vi "F Dwf Enum.vi"(8 "error in (no error)":errorcluster, 10 "pcDevice":i32, 11 "enumfilter":i32) -> (0 "error out":errorcluster, 2 "pcDevice out":i32, 3 "function return":i32)   [LabVIEW 2024, in "Olasdwf.lvlib"]
doc: "DWFAPI int FDwfEnum(ENUMFILTER enumfilter, int *pcDevice);"
uses:
  Olasdwf.lvlib
  Windows/System32/dwf.dll
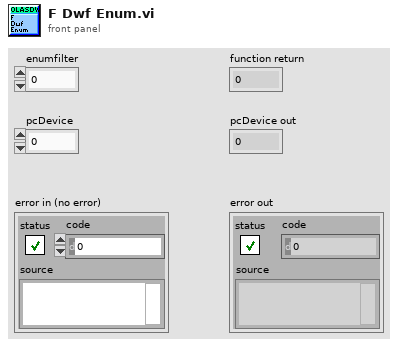
[diagram p1: front panel]
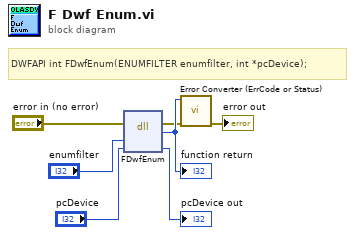
[diagram p0: block diagram]
diagram:
  # "DWFAPI int FDwfEnum(ENUMFILTER enumfilter, int *pcDevice);"
  n1 = dll-call lib="/Windows/System32/dwf.*" fn="FDwfEnum"(error in="error in (no error)", "enumfilter"="enumfilter", "pcDevice"="pcDevice") -> (error out=w2:errorcluster, w7:i32, "pcDevice"=→"pcDevice out":i32)  [unwired: 3 in, 1 out]
  "function return" <- w7
  n2 = call "Error Converter (ErrCode or Status).vi"("error in (no error)"=w2, "error code"=w7) -> ("error out"=→"error out":errorcluster)  [unwired: 9 in]
